vi "testGetConfigEventTest.vi"(8 "error in (no error)":errorcluster) -> (0 "error out":errorcluster)   [LabVIEW 2018]
uses:
  src/SalProcess/SalProcess.lvclass
  <vilib>/addons/_JKI Toolkits/Caraya/classes/Assert/Assert Equal Value and Type_Variant.vi
  <vilib>/addons/_JKI Toolkits/Caraya/classes/Test/Test.lvclass
  <vilib>/addons/_JKI Toolkits/Caraya/classes/Assert/Assert.lvclass
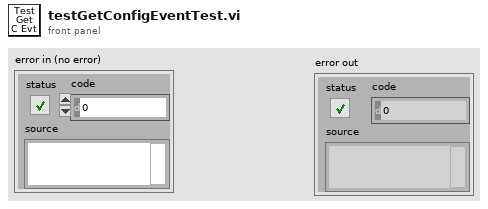
[diagram p1: front panel]
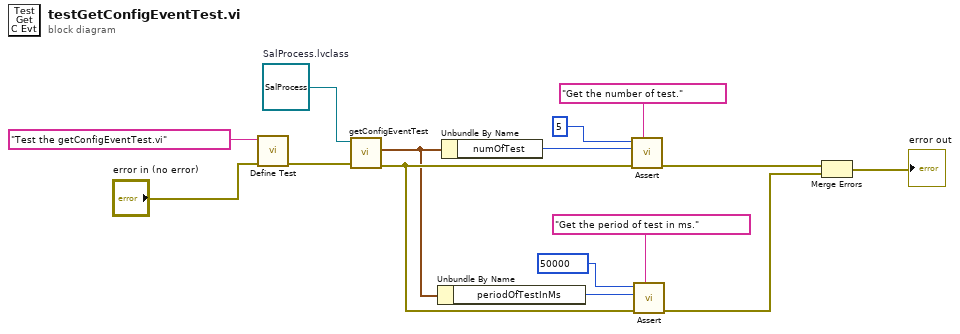
[diagram p0: block diagram]
diagram:
  w12 = refnum<class "SalProcess.lvclass"> refnum  # SalProcess.lvclass
  n1 = call <vilib>:"Define Test.vi"("error in (no error)"="error in (no error)", "Label (VI Title)"="Test the getConfigEventTest.vi") -> ("error out"=w13:errorcluster)  [unwired: 9 in]
  n2 = call "getConfigEventTest.vi"("error in (no error)"=w13, "SalProcess in"=w12) -> ("error out"=w10:errorcluster, "configEventTest"=w9:cluster{"numOfTest":i32, "periodOfTestInMs":u32})  [unwired: 7 in, 1 out]
  n3 = Unbundle By Name(w9) -> ("periodOfTestInMs"=w8:u32)
  n4 = Unbundle By Name(w9) -> ("numOfTest"=w11:i32)
  n5 = call-poly <vilib>:"Assert.vi"("Label"="Get the number of test.", "error in (no error)"=w10, "Y"=w11, "X"=5) -> ("error out"=w3:errorcluster)  [unwired: 7 in]
  n6 = call-poly <vilib>:"Assert.vi"("Label"="Get the period of test in ms.", "error in (no error)"=w10, "Y"=w8, "X"=u32 50000) -> ("error out"=w2:errorcluster)  [unwired: 7 in]
  n7 = Merge Errors(w3, w2) -> (→"error out":errorcluster)
